vi "PhotonPNPResult_Equals.vi"(9 "Other PhotonPNPResult":T1={"IsPresent"=FALSE, "bestReprojErr"=0.0, "altReprojErr"=0.0, "ambiguity"=0.0, "Best"={"TRANSLATION3D"={"X"=0.0, "Y"=0.0, "Z"=0.0}, "ROTATION3D"={"Q_quaternion"={"R"=1.0, "V"=[0.0, 0.0, 0.0]}}, "XF"=FALSE}, "Alt"={"TRANSLATION3D"={"X"=0.0, "Y"=0.0, "Z"=0.0}, "ROTATION3D"={"Q_quaternion"={"R"=1.0, "V"=[0.0, 0.0, 0.0]}}, "XF"=FALSE}} {"Alt"."TRANSLATION3D"."Z" format="%14.3f"; "Alt"."TRANSLATION3D"."Y" format="%14.3f"; "Alt"."TRANSLATION3D"."X" format="%14.3f"; "Best"."TRANSLATION3D"."Z" format="%14.3f"; "Best"."TRANSLATION3D"."Y" format="%14.3f"; "Best"."TRANSLATION3D"."X" format="%14.3f"}, 11 "PhotonPNPResult":T1={"IsPresent"=FALSE, "bestReprojErr"=0.0, "altReprojErr"=0.0, "ambiguity"=0.0, "Best"={"TRANSLATION3D"={"X"=0.0, "Y"=0.0, "Z"=0.0}, "ROTATION3D"={"Q_quaternion"={"R"=1.0, "V"=[0.0, 0.0, 0.0]}}, "XF"=FALSE}, "Alt"={"TRANSLATION3D"={"X"=0.0, "Y"=0.0, "Z"=0.0}, "ROTATION3D"={"Q_quaternion"={"R"=1.0, "V"=[0.0, 0.0, 0.0]}}, "XF"=FALSE}} {"Alt"."TRANSLATION3D"."Z" format="%14.3f"; "Alt"."TRANSLATION3D"."Y" format="%14.3f"; "Alt"."TRANSLATION3D"."X" format="%14.3f"; "Best"."TRANSLATION3D"."Z" format="%14.3f"; "Best"."TRANSLATION3D"."Y" format="%14.3f"; "Best"."TRANSLATION3D"."X" format="%14.3f"}) -> (3 "Equal":bool)   [LabVIEW 2019, in "PhotonVisionLib.lvlib"]
doc: "Determines if two PhotonPNPResult clusters are equal.\n\nInputs:\n - PhotonPNPResult -- PhotonPNPResult cluster.\n - OtherPhotonPNPResult -- OtherPhotonPNPResult cluster.\n\nOutputs:\n - Equal -- Returns TRUE, if both PhotonMultiTargetPNPResult clusters are equal.."
uses:
  PhotonVisionLib.lvlib
  <vilib>/Rock Robotics/WPI/ThirdParty/JAS_Junk/TrajLib/Trajectory_Library.lvlib
  <vilib>/Rock Robotics/WPI/ThirdParty/JAS_Junk/TrajLib/TypeDef/TRANSLATION3D.ctl
  <vilib>/Rock Robotics/WPI/ThirdParty/JAS_Junk/TrajLib/TypeDef/QUATERNION.ctl
  <vilib>/Rock Robotics/WPI/ThirdParty/JAS_Junk/TrajLib/TypeDef/ROTATION3D.ctl
  <vilib>/Rock Robotics/WPI/ThirdParty/JAS_Junk/TrajLib/TypeDef/TRANSFORM3D.ctl
  TypeDef/PhotonPNPResultType.ctl
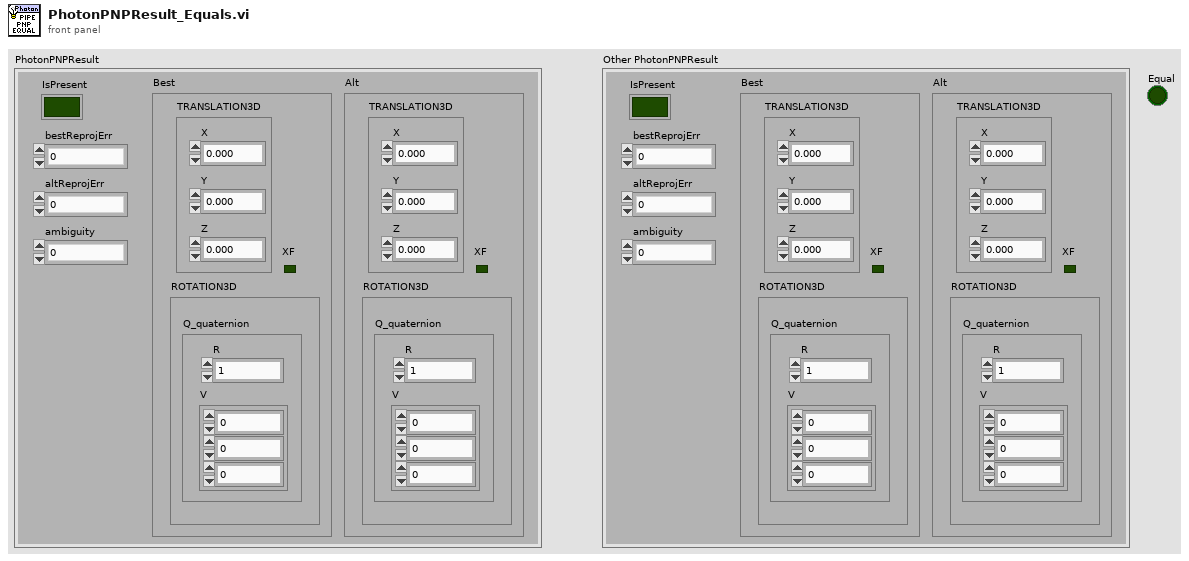
[diagram p1: front panel]
types:
  T1 = typedef "PhotonVisionLib.lvlib/PhotonPNPResultType.ctl" = cluster{"IsPresent":bool, "bestReprojErr":dbl, "altReprojErr":dbl, "ambiguity":dbl, "Best":T2, "Alt":T2}
  T2 = typedef "Trajectory_Library.lvlib/TRANSFORM3D.ctl" = cluster{"TRANSLATION3D":T3, "ROTATION3D":T4, "XF":bool}
  T3 = typedef "Trajectory_Library.lvlib/TRANSLATION3D.ctl" = cluster{"X":dbl, "Y":dbl, "Z":dbl}
  T4 = typedef "Trajectory_Library.lvlib/ROTATION3D.ctl" = cluster{"Q_quaternion":T5}
  T5 = typedef "Trajectory_Library.lvlib/QUATERNION.ctl" = cluster{"R":dbl, "V":dbl[]}
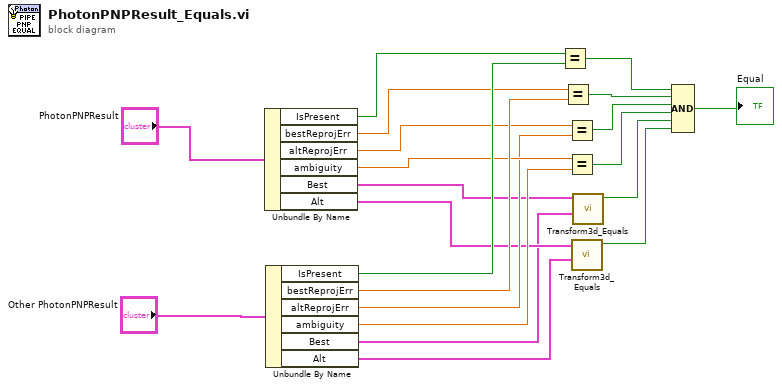
[diagram p0: block diagram]
diagram:
  n1 = Unbundle By Name("PhotonPNPResult") -> ("IsPresent"=w19:bool, "bestReprojErr"=w15:dbl, "altReprojErr"=w8:dbl, "ambiguity"=w7:dbl, "Best"=w4:T2, "Alt"=w3:T2)
  n2 = Unbundle By Name("Other PhotonPNPResult") -> ("IsPresent"=w18:bool, "bestReprojErr"=w17:dbl, "altReprojErr"=w6:dbl, "ambiguity"=w5:dbl, "Best"=w2:T2, "Alt"=w1:T2)
  n3 = Equal?(x=w19, y=w18) -> (x = y?=w14:bool)
  n4 = Equal?(x=w15, y=w17) -> (x = y?=w13:bool)
  n5 = Equal?(x=w8, y=w6) -> (x = y?=w12:bool)
  n6 = Equal?(x=w7, y=w5) -> (x = y?=w11:bool)
  n7 = call <vilib>:"Transform3d_Equals.vi"("otherTransform3d"=w1, "inTransform3d"=w3) -> ("Equals"=w9:bool)  [unwired: 9 in]
  n8 = call <vilib>:"Transform3d_Equals.vi"("otherTransform3d"=w2, "inTransform3d"=w4) -> ("Equals"=w10:bool)  [unwired: 9 in]
  n9 = Compound Arithmetic op=AND(w14, w13, w12, w11, w10, w9) -> (→"Equal":bool)
